vi "Choreo_Util_DefaultDir.vi"(11 "Path in":path) -> (3 "Path Out":path)   [LabVIEW 2019, in "ChoreoLib.lvlib"]
doc: "If given path is relative insert the default data directory. If given path is absolute, pass it through unchanged. The resulting path is always absolute."
uses:
  ChoreoLib.lvlib
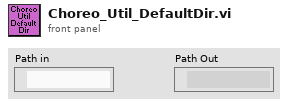
[diagram p1: front panel]
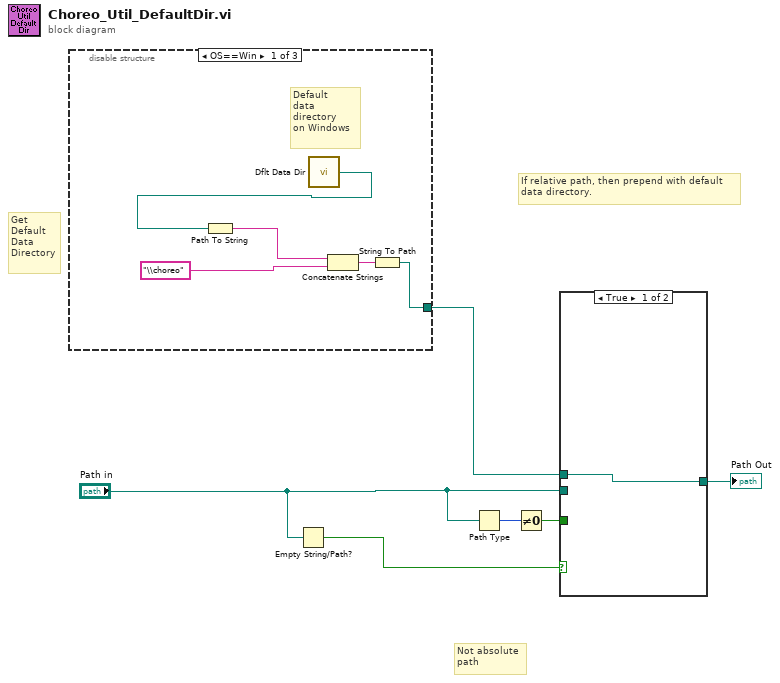
[diagram p0: block diagram]
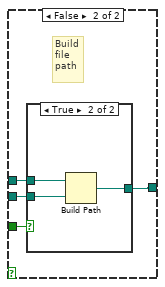
[diagram p2: hidden frame]
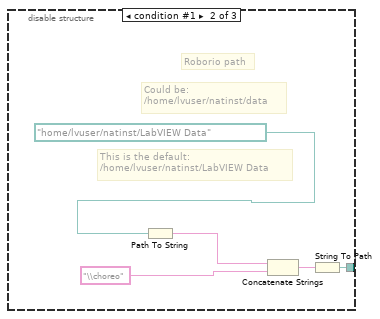
[diagram p4: hidden frame]
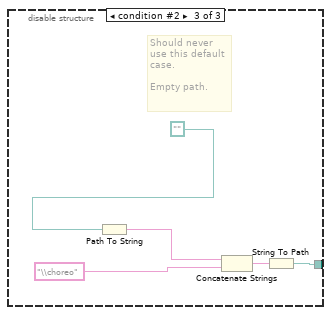
[diagram p5: hidden frame]
diagram:
  # "If relative path, then prepend with default\ndata directory."
  # "Not absolute\npath"
  # "Get\nDefault\nData\nDirectory"
  n1 = disable-structure shown="OS==Win" {
    disable-tunnel: [w7 w15 w17] -> w3
    frame condition #0 (active) {
      # "Default\ndata\ndirectory\non Windows"
      n2 = call <vilib>:"Dflt Data Dir.vi"() -> ("App:Default Data Directory"=w8:path)
      n3 = Path To String(path=w8) -> (string=w10:string)
      n4 = Concatenate Strings(w10, "\\choreo") -> (w11:string)
      n5 = String To Path(string=w11) -> (path=w7:path)
    }
    frame condition #1 {
      # "This is the default:\n/home/lvuser/natinst/LabVIEW Data"
      # "Could be:\n/home/lvuser/natinst/data"
      # "Roborio path"
      n6 = Path To String(path=path "/home/lvuser/natinst/LabVIEW Data") -> (string=w13:string)
      n7 = Concatenate Strings(w13, "\\choreo") -> (w16:string)
      n8 = String To Path(string=w16) -> (path=w15:path)
    }
    frame condition #2 {
      # "Should never\nuse this default\ncase.\n\nEmpty path."
      n9 = Path To String(path=path "") -> (string=w20:string)
      n10 = Concatenate Strings(w20, "\\choreo") -> (w21:string)
      n11 = String To Path(string=w21) -> (path=w17:path)
    }
  }
  n12 = Empty String/Path?(string/path="Path in") -> (empty?=w1:bool)
  n13 = Path Type(1:"Path in") -> (0:w4:i16)
  n14 = Not Equal To 0?(x=w4) -> (x != 0?=w5:bool)
  n15 = case shown="True" w1 {
    tunnel: "Path in" -> [_ w26]
    tunnel: [w22 w25] -> w6
    tunnel: w5 -> [_ w24]
    tunnel: w3 -> [w22 w23]
    frame True {
    }
    frame False {
      # "Build\nfile\npath"
      n16 = case shown="True" w24 {
        tunnel: [w27 w30] -> w25
        tunnel: w23 -> [_ w29]
        tunnel: w26 -> [w27 w28]
        frame False {
        }
        frame True {
          n17 = Build Path(base path=w29, name or relative path=w28) -> (appended path=w30:path)
        }
      }
    }
  }
  "Path Out" <- w6
